vi "Get Velocity ESP.vi"(8 "error in (no error)":errorcluster, 9 "Axis (1)":i32=1 min=1 max=3, 10 "VISA resource name":refnum<visa-resource-name>, 11 "ESP301 in":refnum<class "ESP301.lvclass">) -> (0 "error out":errorcluster, 1 "Velocity (units/s)":dbl format="%.4g", 2 "VISA resource name out":refnum<visa-resource-name>, 3 "ESP301 out":refnum<class "ESP301.lvclass">)   [LabVIEW 2020, in "ESP301.lvclass"]
uses:
  ESP301.lvclass
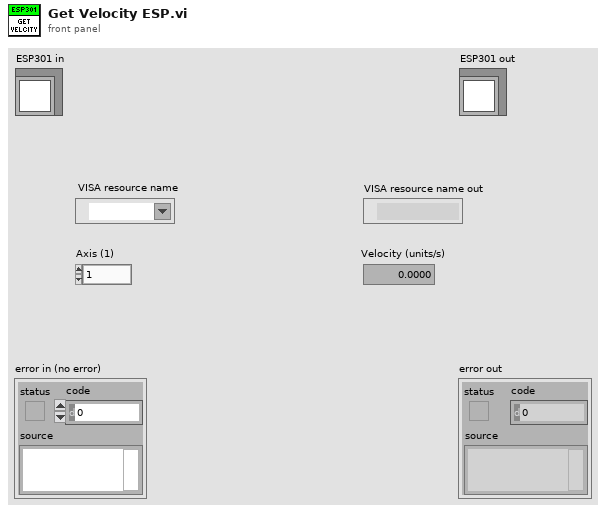
[diagram p1: front panel]
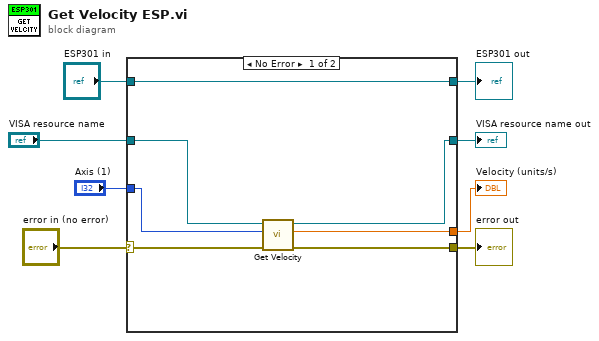
[diagram p0: block diagram]
diagram:
  n1 = case shown="No Error" "error in (no error)" {
    selector: "error in (no error)" -> [w12 w18]
    tunnel: [w11 w18] -> w7
    tunnel: [w15 w17] -> w5
    tunnel: "ESP301 in" -> [w15 w17]
    tunnel: "VISA resource name" -> [w14 w16]
    tunnel: "Axis (1)" -> [w13 _]
    tunnel: [w10 _] -> w2
    tunnel: [w9 w16] -> w1
    frame No Error {
      n2 = call "Get Velocity.vi"("error in (no error)"=w12, "Axis (1)"=w13, "VISA resource name"=w14) -> ("error out"=w11:errorcluster, "Velocity (units/s)"=w10:dbl, "VISA resource name out"=w9:refnum<visa-resource-name>)  [unwired: 2 in]
    }
    frame Error {
    }
  }
  "error out" <- w7
  "ESP301 out" <- w5
  "VISA resource name out" <- w1
  "Velocity (units/s)" <- w2
